vi "write current filter.vi"(8 "error in (no error)":errorcluster, 9 "filterType":u8(ring)=6 items=["K_CHAN_R", "K_CHAN_W", "K_CHAN_RW", "K_CHAN_VOLT", "K_CHAN_FAULT", "K_ALL", "K_CUSTOM", "K_CHAN_R_VIS", "K_CHAN_W_VIS", "K_CHAN_RW_VIS", "K_CHAN_VOLT_VIS", "K_CHAN_FAULT_VIS", "K_WAVE", "K_WAVE_VIS", "K_WAVE_DBL", "K_WAVE_CDB", "K_WAVE_DBL_VIS", "K_WAVE_CDB_VIS"], 10 "Filter":refnum<k24>, 11 "alias-tree in":refnum<class "alias-tree.lvclass">) -> (0 "error out":errorcluster, 3 "alias-tree out":refnum<class "alias-tree.lvclass">)   [LabVIEW 2017, in "vs-tree-utility.lvlib" / "alias-tree.lvclass"]
uses:
  alias-tree.lvclass
  NationalInstruments.VeriStand.SystemStorage
  NationalInstruments.VeriStand.SystemStorageUI
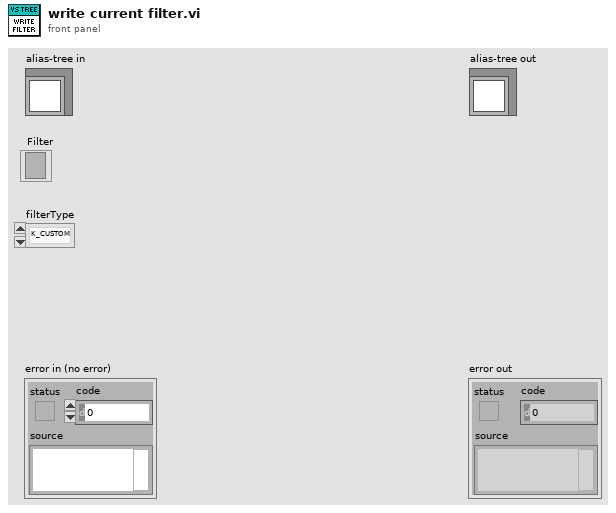
[diagram p1: front panel]
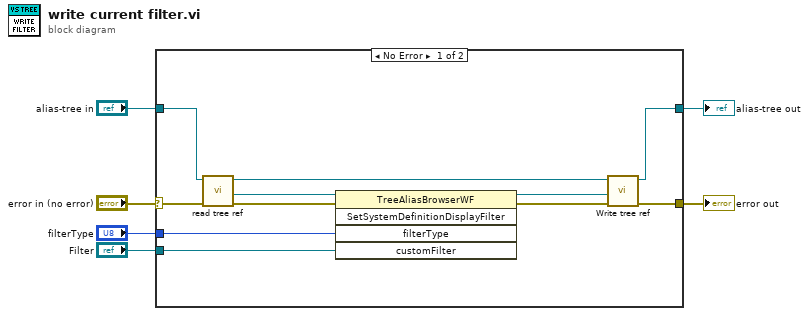
[diagram p0: block diagram]
diagram:
  n1 = case shown="No Error" "error in (no error)" {
    selector: "error in (no error)" -> [w17 w19]
    tunnel: [w13 w19] -> w5
    tunnel: [w9 w18] -> w3
    tunnel: "alias-tree in" -> [w11 w18]
    tunnel: "Filter" -> [w8 _]
    tunnel: "filterType" -> [w7 _]
    frame No Error {
      n2 = call-dynamic "read tree ref.vi"("error in (no error)"=w17, "alias-tree in"=w11) -> ("error out"=w16:errorcluster, "tree ref"=w15:refnum<k24>, "alias-tree out"=w10:refnum<class "alias-tree.lvclass">)  [unwired: 7 in]
      n3 = invoke class="TreeAliasBrowserWF" method="SetSystemDefinitionDisplayFilter"(reference=w15, error in=w16, "filterType"=w7, "customFilter"=w8) -> (reference out=w12:refnum<k24>, error out=w14:errorcluster)  [unwired: 1 in, 3 out]
      n4 = call-dynamic "Write tree ref.vi"("error in (no error)"=w14, "tree ref"=w12, "alias-tree in"=w10) -> ("error out"=w13:errorcluster, "alias-tree out"=w9:refnum<class "alias-tree.lvclass">)  [unwired: 7 in]
    }
    frame Error {
    }
  }
  "error out" <- w5
  "alias-tree out" <- w3
